vi "Teleop.vi"(10 "Match Info":T1={"Autonomous Elapsed Seconds"=0.0, "TeleOp Elapsed Seconds"=0.0, "Disabled Elapsed Seconds"=0.0, "Visited Autonomous"=FALSE, "Visited TeleOp"=FALSE, "Visited Disabled"=FALSE, "Autonomous Settings"={"Autonomous Style"=enum."Independent", "VI Refnum"=refnum}}, 11 "Call Context":T2) -> ()   [LabVIEW 2012]
doc: "This VI is called for each TeleOp packet received from the DS where the robot is not disabled. It is often used to read from the joysticks and update I/O or to update setpoints for timed control loops. It should complete and return within 20 milliseconds or it may miss DS packets."
uses:
  <vilib>/Rock Robotics/WPI/DriverStation/WPI_DriverStationDerivedRobotMode.ctl
  <vilib>/Rock Robotics/WPI/DriverStation/WPI_DriverStationMatch Info.ctl
  <vilib>/Rock Robotics/WPI/Solenoid/WPI_SolenoidValue.ctl
  Robot Global Data.vi
  Autonomous_Routine_Global.vi
  <vilib>/Rock Robotics/WPI/Solenoid/WPI_SolenoidSetEnum.vi
  <vilib>/Rock Robotics/WPI/RobotDrive/WPI_RobotDriveMecanumDrive_Cartesian.vi
  <vilib>/Rock Robotics/WPI/RobotDrive/WPI_RobotDriveGetSetRefNum.vi
  <vilib>/Rock Robotics/WPI/Joystick/WPI_JoystickGetSetRefNum.vi
panel:
  out "error out":errorcluster
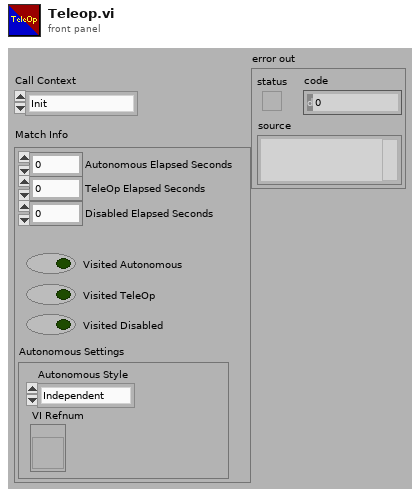
[diagram p1: front panel]
types:
  T1 = typedef "WPI_DriverStationMatch Info.ctl" = cluster{"Autonomous Elapsed Seconds":dbl, "TeleOp Elapsed Seconds":dbl, "Disabled Elapsed Seconds":dbl, "Visited Autonomous":bool, "Visited TeleOp":bool, "Visited Disabled":bool, "Autonomous Settings":cluster{"Autonomous Style":enum16{"Iterative", "Independent"}, "VI Refnum":refnum<vi>}}
  T2 = typedef "WPI_DriverStationDerivedRobotMode.ctl" = enum16{"Init", "Execute", "Stop"}
  T3 = typedef "WPI_SolenoidValue.ctl" = enum16{"Off", "On", "Forward", "Reverse"}
  T4 = typedef "WPI_JoystickDevRef.ctl" = cluster{"Device":T5}
  T5 = typedef "WPI_JoystickDeviceEnum.ctl" = enum16{"USB 1", "USB 2", "USB 3", "USB 4", "Kinect 1", "Kinect 2"}
  T6 = typedef "WPI_JoystickButtonState.ctl" = cluster{"Button 1":bool, "Button 2":bool, "Button 3":bool, "Button 4":bool, "Button 5":bool, "Button 6":bool, "Button 7":bool, "Button 8":bool, "Button 9":bool, "Button 10":bool, "Button 11":bool, "Button 12":bool}
  T7 = cluster{"axis 1 (x)":dbl, "axis 2 (y)":dbl, "axis 3 (throttle)":dbl, "axis 4":dbl, "axis 5":dbl, "axis 6":dbl}
  T8 = typedef "WPI_MotorControlDeviceRef.ctl" = cluster{"DeviceStatus":errorcluster, "Type":enum16{"PWM", "CAN"}, "PWM":cluster{"Digital Module":T9, "PWM Channel":T10, "DeadBand":T11}, "CAN":cluster{"Device Number":u8, "Control Mode":T12, "Semaphore":T13, "Max Vout":dbl}, "Invert":bool, "TransformRef":T14, "InvTransformRef":T14}
  T9 = typedef "FPGA_TypedefDigitalModule.ctl" = enum16{"Digital Module 1", "Digital Module 2"}
  T10 = typedef "FPGA_DIOPWMChannel.ctl" = enum8{"PWM 1", "PWM 2", "PWM 3", "PWM 4", "PWM 5", "PWM 6", "PWM 7", "PWM 8", "PWM 9", "PWM 10", "Invalid"}
  T11 = typedef "WPI_PWMDeadband.ctl" = cluster{"Name":string, "maxPositivePwm":i32, "minPositivePwm":i32, "centerPwm":i32, "maxNegativePwm":i32, "minNegativePwm":i32, "angularRange":u16}
  T12 = typedef "WPI_CANJaguar_ControlMode.ctl" = enum8{"Percent VBus", "Current", "Speed", "Position", "Voltage"}
  T13 = typedef "Semaphore RefNum" = refnum<k1>
  T14 = typedef "WPI_PWMTransform_ConPane.ctl" = refnum<vi>
  T15 = typedef "WPI_SolenoidDevRef.ctl" = cluster{"DevStatus":errorcluster, "Solenoid Module":T16, "Forward Solenoid Channel":T17, "Reverse Solenoid Channel":T17}
  T16 = typedef "FPGA_TypedefSolenoidModule.ctl" = enum16{"Solenoid Module 1", "Solenoid Module 2"}
  T17 = typedef "WPI_SolenoidChannel.ctl" = enum8{"Solenoid 1", "Solenoid 2", "Solenoid 3", "Solenoid 4", "Solenoid 5", "Solenoid 6", "Solenoid 7", "Solenoid 8", "Invalid"}
  T18 = typedef "WPI_RobotDriveDevRef.ctl" = cluster{"DevStatus":errorcluster, "Motors[]":T8[], "Square Inputs":bool, "Max Output":dbl, "Isochronous":bool}
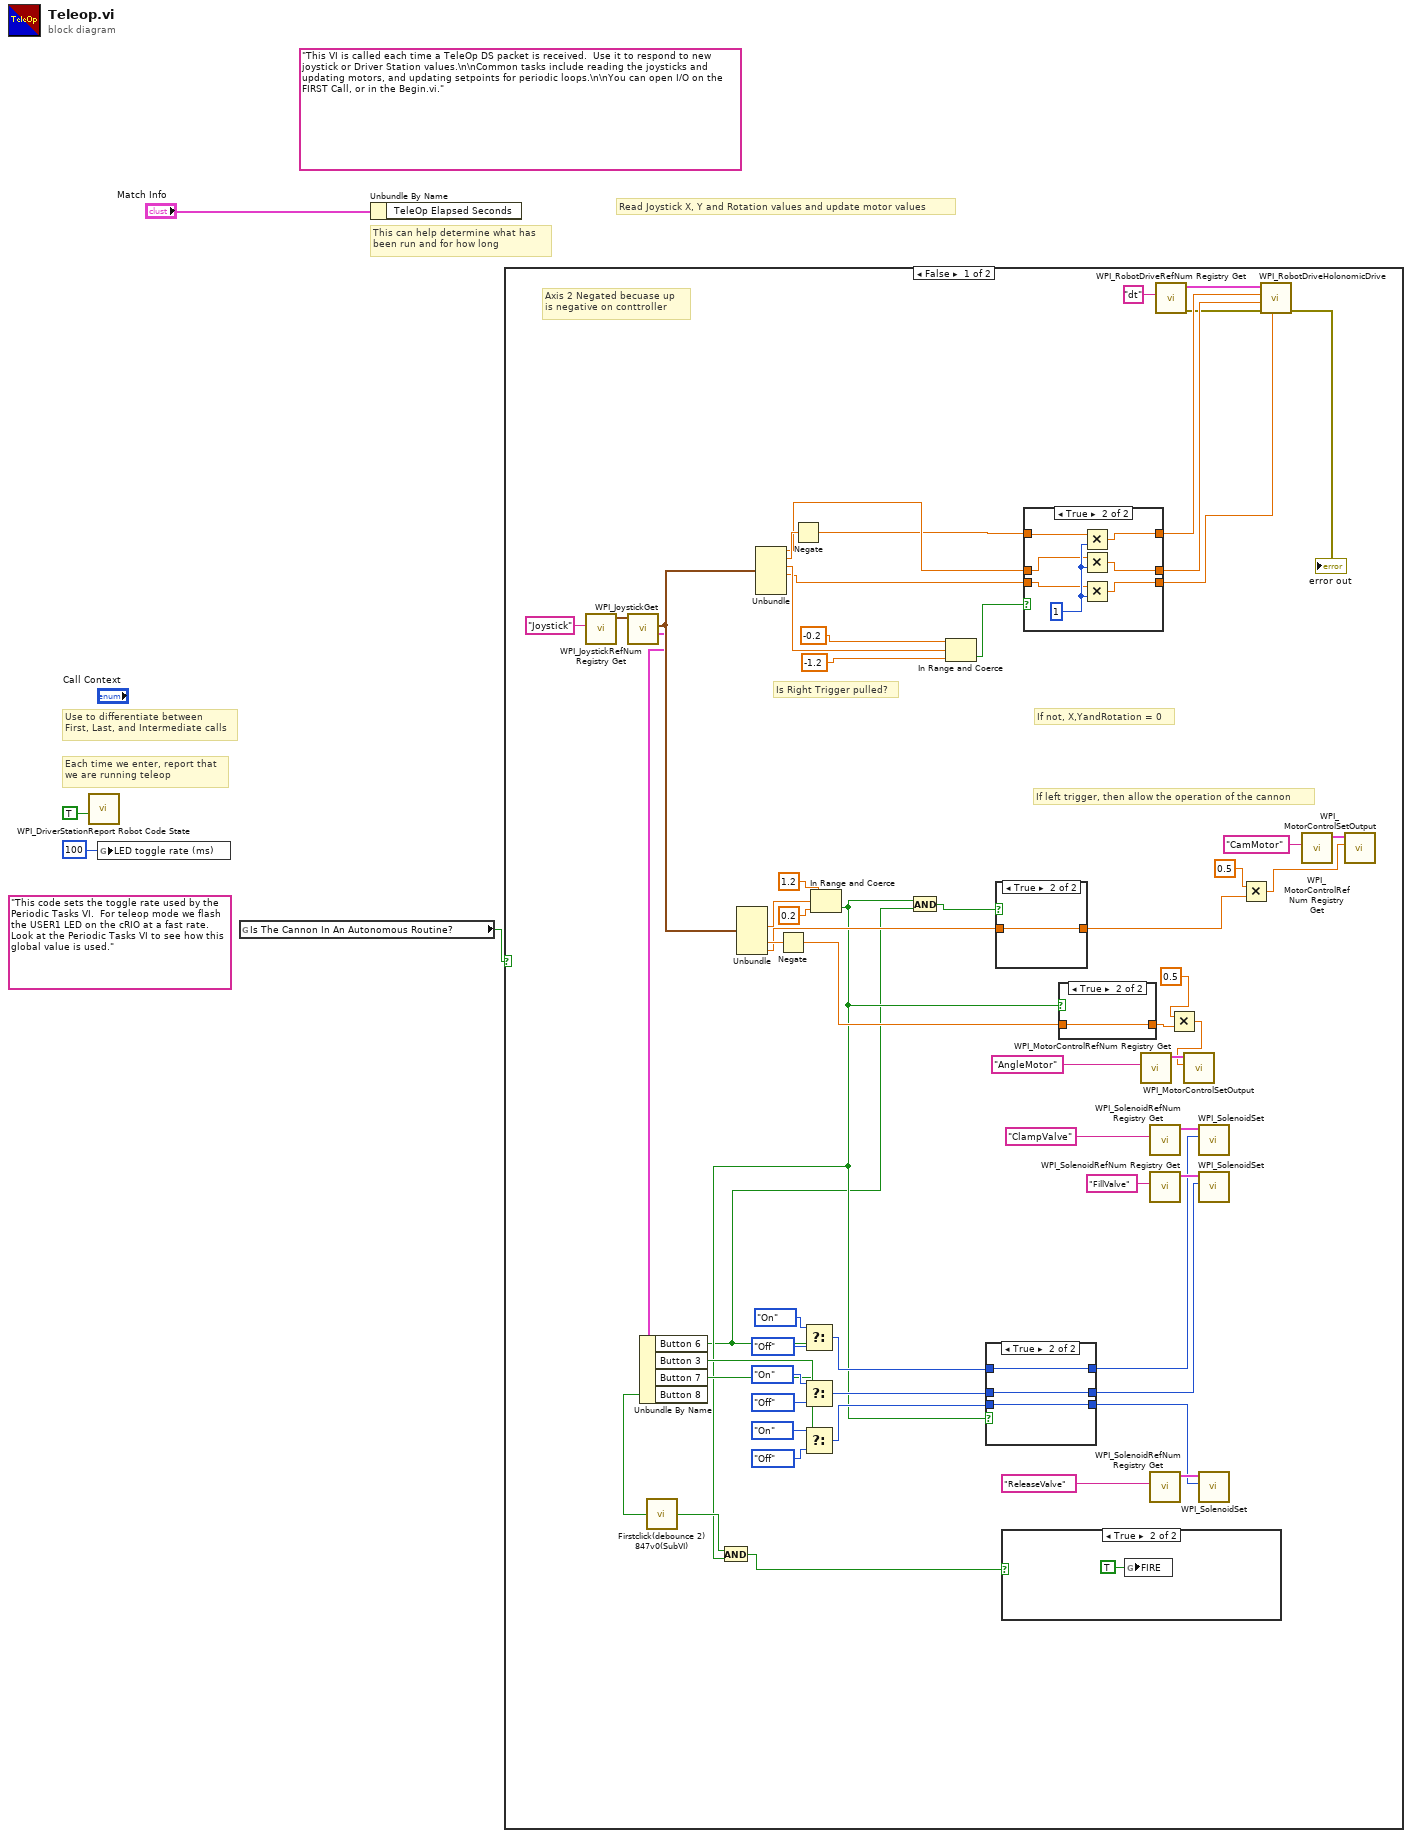
[diagram p0: block diagram]
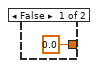
[diagram p2: hidden frame]
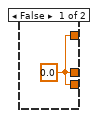
[diagram p3: hidden frame]
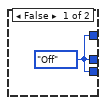
[diagram p5: hidden frame]
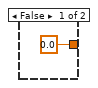
[diagram p6: hidden frame]
diagram:
  (unwired) "This code sets the toggle rate used by the Periodic Tasks VI.  For teleop mode we flash the USER1 LED on the cRIO at a fast rate.  Look at the Periodic Tasks VI to see how this global value is used."
  (unwired) "This VI is called each time a TeleOp DS packet is received.  Use it to respond to new joystick or Driver Station values.\n\nCommon tasks include reading the joysticks and updating motors, and updating setpoints for periodic loops.\n\nYou can open I/O on the FIRST Call, or in the Begin.vi."
  # "Each time we enter, report that\nwe are running teleop"
  # "Use to differentiate between\nFirst, Last, and Intermediate calls"
  # "This can help determine what has\nbeen run and for how long"
  # "Read Joystick X, Y and Rotation values and update motor values"
  n1 = call <vilib>:"WPI_DriverStationReport Robot Code State.vi"("TeleOp"=TRUE ("Autonomous")) -> ()  [unwired: 10 in, 1 out]
  n2 = global write "Robot Global Data.vi" "LED toggle rate (ms)"(u32 100 ("LED ms toggle rate")) -> ()
  n3 = global read "Autonomous_Routine_Global.vi" "Is The Cannon In An Autonomous Routine?"() -> (w1:bool)
  n4 = Unbundle By Name("Match Info") -> ()  [unwired: 1 out]
  n5 = case shown="False" w1 {
    frame False {
      # "Axis 2 Negated becuase up \nis negative on conttroller"
      # "If left trigger, then allow the operation of the cannon"
      # "If not, X,YandRotation = 0"
      # "Is Right Trigger pulled?"
      n6 = call <vilib>:"WPI_JoystickRefNum Registry Get.vi"("refnum name"="Joystick") -> ("JoystickDevRef"=w64:T4)  [unwired: 9 in, 1 out]
      n7 = call <vilib>:"WPI_JoystickGet.vi"("JoystickDevRef"=w64) -> ("Buttons"=w53:T6, "Axes"=w59:T7)  [unwired: 4 in, 1 out]
      n8 = Unbundle By Name(w53) -> ("Button 6"=w11:bool, "Button 3"=w34:bool, "Button 7"=w33:bool, "Button 8"=w32:bool)
      n9 = call "Firstclick(debounce 2) 847v0(SubVI).vi"("Input"=w32) -> ("output"=w16:bool)
      n10 = Unbundle(w59) -> ("axis 3 (throttle)"=w58:dbl, "axis 5"=w57:dbl, "axis 6"=w54:dbl)  [unwired: 3 out]
      n11 = Unbundle(w59) -> ("axis 1 (x)"=w7:dbl, "axis 2 (y)"=w22:dbl, "axis 3 (throttle)"=w27:dbl, "axis 4"=w5:dbl)  [unwired: 2 out]
      n12 = Negate(x=w57) -> (-x=w14:dbl)
      n13 = Negate(x=w22) -> (-x=w6:dbl)
      n14 = Select(t=WPI_SolenoidValue."On" ("Value"), s=w11, f=WPI_SolenoidValue."Off" ("Value")) -> (s? t:f=w44:T3)
      n15 = Select(t=WPI_SolenoidValue."On" ("Value"), s=w34, f=WPI_SolenoidValue."Off" ("Value")) -> (s? t:f=w45:T3)
      n16 = Select(t=WPI_SolenoidValue."On" ("Value"), s=w33, f=WPI_SolenoidValue."Off" ("Value")) -> (s? t:f=w46:T3)
      n17 = In Range and Coerce(upper limit=1.2, x=w58, lower limit=0.2) -> (In Range?=w12:bool)  [unwired: 1 out]
      n18 = And(x=w16, y=w12) -> (x .and. y?=w15:bool)
      n19 = And(x=w12, y=w11) -> (x .and. y?=w13:bool)
      n20 = In Range and Coerce(upper limit=-0.2, x=w27, lower limit=-1.2) -> (In Range?=w26:bool)  [unwired: 1 out]
      n21 = case shown="True" w12 {
        tunnel: w46 -> [_ w78]
        tunnel: w45 -> [_ w79]
        tunnel: w44 -> [_ w80]
        tunnel: [w77 w80] -> w37
        tunnel: [w77 w79] -> w36
        tunnel: [w77 w78] -> w35
        frame False {
          w77 = WPI_SolenoidValue."Off" ("Value")
        }
        frame True {
        }
      }
      n22 = case shown="True" w13 {
        tunnel: w54 -> [_ w82]
        tunnel: [0.0 w82] -> w19
        frame False {
        }
        frame True {
        }
      }
      n23 = case shown="True" w15 {
        frame False {
        }
        frame True {
          n24 = global write "Autonomous_Routine_Global.vi" "FIRE"(TRUE ("FIRE")) -> ()
        }
      }
      n25 = case shown="True" w26 {
        tunnel: w7 -> [_ w70]
        tunnel: w6 -> [_ w71]
        tunnel: w5 -> [_ w69]
        tunnel: [w68 w72] -> w25
        tunnel: [w68 w73] -> w24
        tunnel: [w68 w74] -> w23
        frame False {
          w68 = 0.0 ("axis 1 (x)")
        }
        frame True {
          w75 = 1
          n26 = Multiply(x=w71, y=w75) -> (x*y=w74:dbl)
          n27 = Multiply(x=w70, y=w75) -> (x*y=w73:dbl)
          n28 = Multiply(x=w69, y=w75) -> (x*y=w72:dbl)
        }
      }
      n29 = case shown="True" w12 {
        tunnel: w14 -> [_ w67]
        tunnel: [0.0 w67] -> w9
        frame False {
        }
        frame True {
        }
      }
      n30 = call <vilib>:"WPI_MotorControlRefNum Registry Get.vi"("refnum name"="AngleMotor") -> ("MotorControlDevRef"=w63:T8)  [unwired: 9 in, 1 out]
      n31 = call <vilib>:"WPI_SolenoidRefNum Registry Get.vi"("refnum name"="ClampValve") -> ("SolenoidDevRef"=w42:T15)  [unwired: 9 in, 1 out]
      n32 = call <vilib>:"WPI_SolenoidRefNum Registry Get.vi"("refnum name"="FillValve") -> ("SolenoidDevRef"=w41:T15)  [unwired: 9 in, 1 out]
      n33 = call <vilib>:"WPI_SolenoidRefNum Registry Get.vi"("refnum name"="ReleaseValve") -> ("SolenoidDevRef"=w38:T15)  [unwired: 9 in, 1 out]
      n34 = call <vilib>:"WPI_RobotDriveRefNum Registry Get.vi"("refnum name"="dt") -> ("error out"=w21:errorcluster, "RobotDriveDevRef"=w31:T18)  [unwired: 9 in]
      n35 = Multiply(x=0.5, y=w9) -> (x*y=w8:dbl)
      n36 = call <vilib>:"WPI_MotorControlSetOutput.vi"("Output"=w8, "MotorControlDevRef"=w63) -> ()  [unwired: 7 in, 3 out]
      n37 = call-poly <vilib>:"WPI_SolenoidSet.vi"("Value"=w37, "SolenoidDevRef"=w42) -> ()  [unwired: 8 in, 2 out]
      n38 = call-poly <vilib>:"WPI_SolenoidSet.vi"("Value"=w36, "SolenoidDevRef"=w41) -> ()  [unwired: 8 in, 2 out]
      n39 = call-poly <vilib>:"WPI_SolenoidSet.vi"("Value"=w35, "SolenoidDevRef"=w38) -> ()  [unwired: 8 in, 2 out]
      n40 = Multiply(x=0.5, y=w19) -> (x*y=w17:dbl)
      n41 = call-poly <vilib>:"WPI_RobotDriveHolonomicDrive.vi"("Rotation"=w25, "error in (no error)"=w21, "Y"=w24, "X"=w23, "RobotDriveDevRef"=w31) -> ("error out"=→"error out":errorcluster)  [unwired: 4 in, 2 out]
      n42 = call <vilib>:"WPI_MotorControlRefNum Registry Get.vi"("refnum name"="CamMotor") -> ("MotorControlDevRef"=w55:T8)  [unwired: 9 in, 1 out]
      n43 = call <vilib>:"WPI_MotorControlSetOutput.vi"("Output"=w17, "MotorControlDevRef"=w55) -> ()  [unwired: 7 in, 3 out]
    }
    frame True {
    }
  }
